vi "get rx gain.vi"(8 "error in":errorcluster, 11 "MultiUsrp in":refnum<class "MultiUsrp.lvclass">) -> (0 "error out":errorcluster, 2 "gain":dbl, 3 "MultiUsrp out":refnum<class "MultiUsrp.lvclass">)   [LabVIEW 2023, in "uhd.lvlib" / "MultiUsrp.lvclass"]
uses:
  <userlib>/uhd/MultiUsrp/MultiUsrp.lvclass
  <userlib>/uhd/MultiUsrp/MultiUsrp.lvclass/MultiUsrp.ctl
  <userlib>/uhd/uhd.lvlib
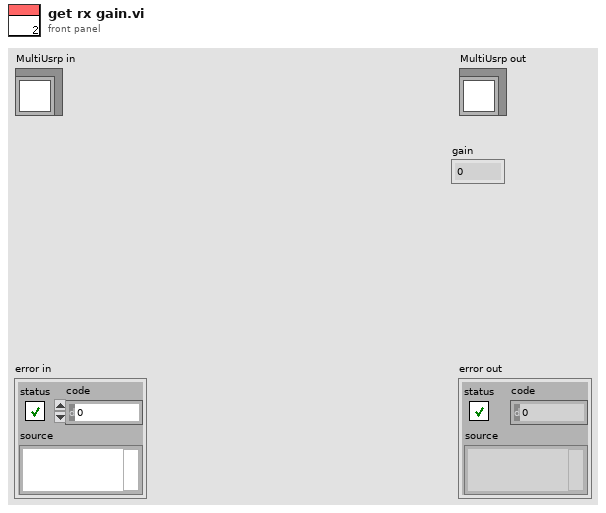
[diagram p1: front panel]
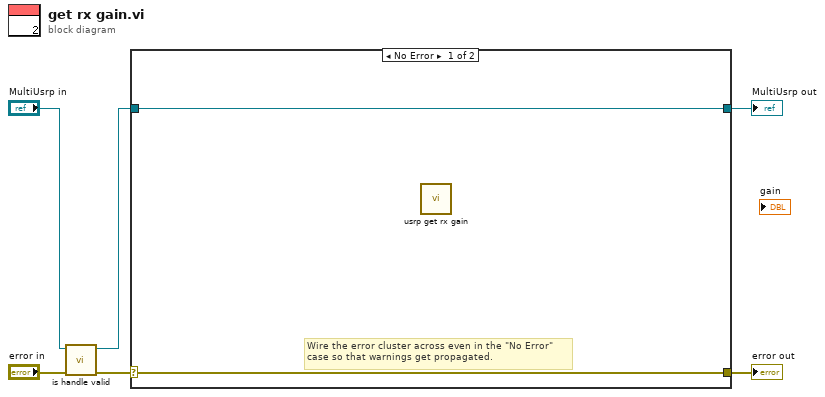
[diagram p0: block diagram]
diagram:
  n1 = call <userlib>:"is handle valid.vi"("error in (no error)"="error in", "MultiUsrp in"="MultiUsrp in") -> ("error out"=w3:errorcluster, "MultiUsrp out"=w1:refnum<class "MultiUsrp.lvclass">)  [unwired: 8 in]
  n2 = case shown="No Error" w3 {
    selector: w3 -> [w7 w10]
    tunnel: [w7 w10] -> w6
    tunnel: [w8 w9] -> w5
    tunnel: w1 -> [w8 w9]
    frame No Error {
      # "Wire the error cluster across even in the \"No Error\"\ncase so that warnings get propagated."
      n3 = call <userlib>:"usrp get rx gain.vi"() -> ()  [unwired: 8 in, 4 out]
    }
    frame Error {
    }
  }
  "error out" <- w6
  "MultiUsrp out" <- w5
